vi "svfa_Spectral Compensation for Other Tones.vi"(7 "other tones' information":T2(array[cluster]) {"phase [degree]" format="%.2f"; "amplitude" format="%.2f"; "frequency" format="%.2f"}, 9 "window size":i32, 10 "window":T1(ring), 11 "FFT spectrum":cluster{"f0":dbl, "df":dbl, "spectrum":cdb[]}={"f0"=0.0, "df"=1.0, "spectrum"=[]} {"spectrum" format="%.2f"; "df" format="%.2f"; "f0" format="%.2f"}) -> (3 "compensated FFT spectrum":cluster{"f0":dbl, "df":dbl, "spectrum":cdb[]}={"f0"=0.0, "df"=1.0, "spectrum"=[]} {"spectrum" format="%.2f"; "df" format="%.2f"; "f0" format="%.2f"})   [LabVIEW 2017]
uses:
  <vilib>/addons/_NISVFA/_Spectrum Processing/subVIs/svfa_Window Frequency Response (double array).vi
  <vilib>/addons/_NISVFA/_Spectrum Processing/subVIs/svfa_Rect Window Frequency Response.vi
  <vilib>/addons/_NISVFA/_Spectrum Processing/subVIs/svfa_Cosine Window Coefficients.vi
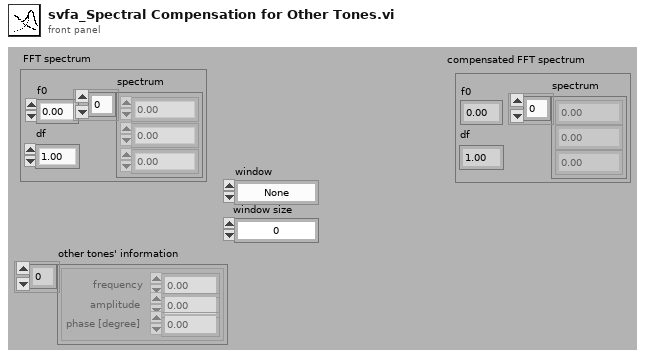
[diagram p1: front panel]
types:
  T1 = enum16{"None ", "Hanning", "Hamming", "Blackman-Harris", "Exact Blackman", "Blackman", "Flat Top", "4 Term B-Harris ", "7 Term B-Harris", "Low Sidelobe"}
  T2 = cluster{"frequency":dbl, "amplitude":dbl, "phase [degree]":dbl}[]
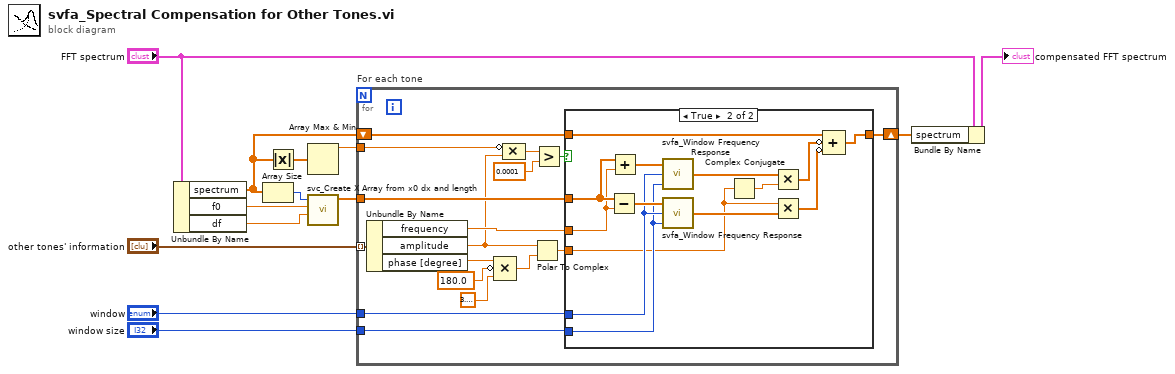
[diagram p0: block diagram]
diagram:
  n1 = Unbundle By Name("FFT spectrum") -> ("spectrum"=w3:cdb[], "f0"=w7:dbl, "df"=w6:dbl)
  n2 = Array Size(array=w3) -> (size(s)=w5:i32)
  n3 = Absolute Value(x=w3) -> (abs(x)=w11:dbl[])
  n4 = Array Max & Min(array=w11) -> (max value=w10:dbl)  [unwired: 3 out]
  n5 = call <vilib>:"svc_Create X Array from x0 dx and length.vi"("dx"=w6, "x0"=w7, "length"=w5) -> ("X"=w2:dbl[])  [unwired: 8 in]
  n6 = for "For each tone" {
    tunnel: "other tones' information" -> [w30] mode=indexing
    tunnel: w2 -> [w27]
    shift-right: [w28] -> w4
    shift-left: w3 -> [w29]
    tunnel: "window" -> [w24]
    tunnel: "window size" -> [w23]
    tunnel: w10 -> [w22]
    n7 = Unbundle By Name(w30) -> ("frequency"=w26:dbl, "amplitude"=w16:dbl, "phase [degree]"=w15:dbl)
    n8 = Compound Arithmetic op=MULTIPLY(w15, invert 180.0 ("y"), 3.141592653589793) -> (w19:dbl)
    n9 = Compound Arithmetic op=MULTIPLY(invert w22, w16) -> (w21:dbl)
    n10 = Polar To Complex(1:w19, 2:w16) -> (0:w14:cdb)
    n11 = Greater?(x=w21, y=0.0001) -> (0:w25:bool)
    n12 = case shown="True" w25 {
      tunnel: w26 -> [_ w36]
      tunnel: w29 -> [w31 w33]
      tunnel: [w31 w41] -> w28
      tunnel: w27 -> [_ w37]
      tunnel: w24 -> [_ w35]
      tunnel: w23 -> [_ w34]
      tunnel: w14 -> [_ w32]
      frame False {
      }
      frame True {
        n13 = Subtract(x=w37, y=w36) -> (x-y=w44:dbl[])
        n14 = Add(x=w37, y=w36) -> (x+y=w45:dbl[])
        n15 = call-poly <vilib>:"svfa_Window Frequency Response.vi"("N (window length)"=w34, "window"=w35, "f(normalized)"=w45) -> ("H(f)"=w43:cdb[])
        n16 = call-poly <vilib>:"svfa_Window Frequency Response.vi"("N (window length)"=w34, "window"=w35, "f(normalized)"=w44) -> ("H(f)"=w42:cdb[])
        n17 = Complex Conjugate(1:w32) -> (0:w39:cdb)
        n18 = Multiply(x=w43, y=w39) -> (x*y=w40:cdb[])
        n19 = Multiply(x=w32, y=w42) -> (x*y=w38:cdb[])
        n20 = Compound Arithmetic op=ADD(w33, invert w40, invert w38) -> (w41:cdb[])
      }
    }
  }
  n21 = Bundle By Name(cluster="FFT spectrum", "spectrum"=w4) -> (→"compensated FFT spectrum":cluster{"f0":dbl, "df":dbl, "spectrum":cdb[]})
